vi "Parse Auto Data.vi"(10 "Is Blue Alliance?":bool=TRUE, 11 "path":path) -> (1 "Zero Velocity?":bool[](array[boolean]), 2 "Velocities":T3[](array[typedef]), 3 "Positions":cluster{"x":dbl, "y":dbl, "th":dbl}[](array[cluster]), 5 "Commands out":cluster{"Time (s)":dbl, T1, bool}[](array[cluster]), 7 "Overall":cluster{"Time (s)":dbl, "Distance (ft)":dbl})   [LabVIEW 2023]
uses:
  swerve/Type Definitions/Data/Robot Velocities.ctl
  bordeaux-pathinator/Bordeaux/Types/Single Cmd Info.ctl
  <vilib>/picture/picture.llb/imagedata.ctl
  <vilib>/Analysis/coordinate.llb/2D Cartesian Coordinate Rotation (Scalar).vi
  <vilib>/Rock Robotics/Network Tables/NT Read Boolean.vi
  <vilib>/Analysis/NI_AALPro.lvlib
panel:
  out "XY Graph":cluster{dbl[], dbl[]}[](graph)
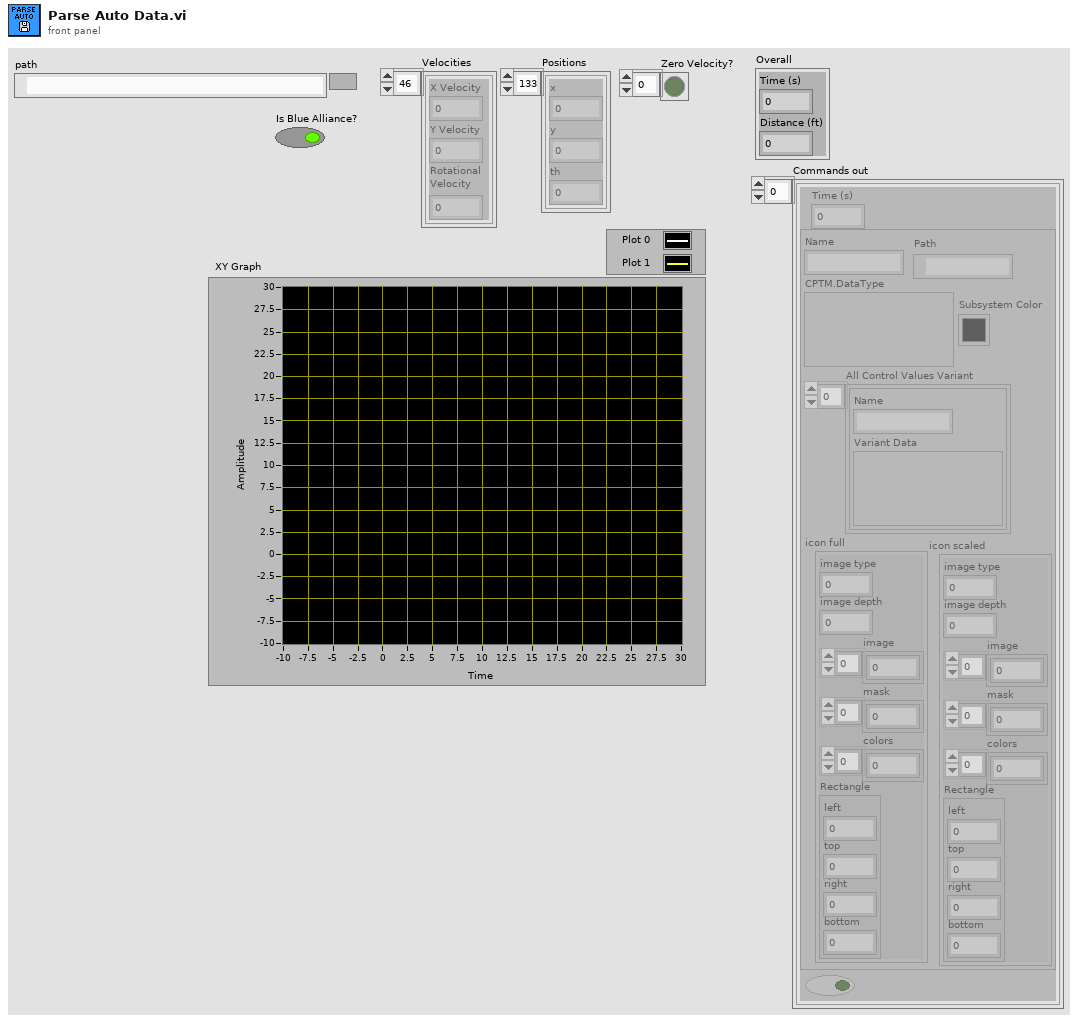
[diagram p1: front panel]
types:
  T1 = typedef "Single Cmd Info.ctl" = cluster{"Name":string, "CPTM.DataType":variant, "All Control Values Variant":cluster{"Name":string, "Variant Data":variant}[], "icon full":T2, "icon scaled":T2, "Path":path, "Subsystem Color":u32}
  T2 = typedef "imagedata.ctl" = cluster{"image type":i32, "image depth":i32, "image":u8[], "mask":u8[], "colors":u32[], "Rectangle":cluster{"left":i16, "top":i16, "right":i16, "bottom":i16}}
  T3 = typedef "Robot Velocities.ctl" = cluster{"X Velocity":dbl, "Y Velocity":dbl, "Rotational \nVelocity":dbl}
  T4 = typedef "Trajectory Data.ctl" = cluster{"Segment Name":string, "Type":T5, "Traj Pos Points":cluster{"x":dbl, "y":dbl, "th":dbl}[], "Traj Vel Points":cluster{"V":dbl, "Omega":dbl, "V vector":cluster{"y":dbl, "x":dbl}}[], "Accel Index":i32, "Decel Index":i32}[]
  T5 = typedef "Segment Type.ctl" = enum16{"Accel Straight", "Const Straight", "Blend", "Circle", "Bezier"}
  T6 = cluster{"V":dbl, "Omega":dbl, "V vector":cluster{"y":dbl, "x":dbl}}[]
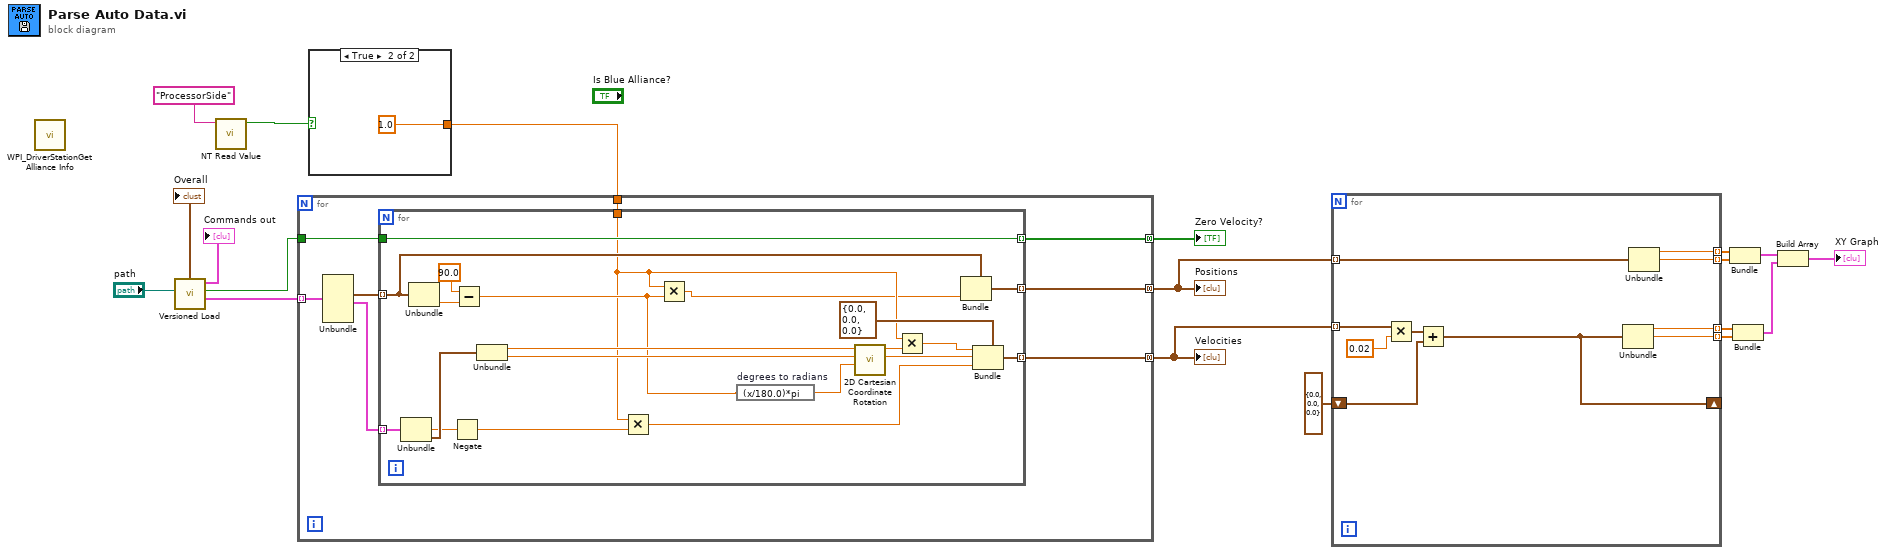
[diagram p0: block diagram]
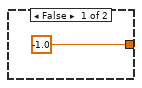
[diagram p2: hidden frame]
diagram:
  n1 = call <vilib>:"WPI_DriverStationGet Alliance Info.vi"() -> ()  [unwired: 6 in, 6 out]
  n2 = call "Versioned Load.vi"("path"="path") -> ("Trajectory Data"=w19:T4, "Zero V"=w17:bool, "Commands out"=→"Commands out":cluster{"Time (s)":dbl, T1, bool}[], "Overall"=→"Overall":cluster{"Time (s)":dbl, "Distance (ft)":dbl})  [unwired: 3 in, 4 out]
  n3 = call-poly <vilib>:"NT Read Value.vi"("name"="ProcessorSide") -> ("value"=w2:bool)  [unwired: 8 in, 2 out]
  n4 = case shown="True" w2 {
    tunnel: [-1.0 1.0] -> w18
    frame False {
    }
    frame True {
    }
  }
  n5 = for {
    tunnel: w19 -> [w29] mode=indexing
    tunnel: [w26] -> w14 mode=concatenating
    tunnel: w18 -> [w25]
    tunnel: [w22] -> w13 mode=concatenating
    tunnel: w17 -> [w24]
    tunnel: [w23] -> w16 mode=concatenating
    n6 = Unbundle(w29) -> ("Traj Pos Points"=w28:cluster{"x":dbl, "y":dbl, "th":dbl}[], "Traj Vel Points"=w27:T6)  [unwired: 4 out]
    n7 = for {
      tunnel: w28 -> [w48] mode=indexing
      tunnel: w27 -> [w46] mode=indexing
      tunnel: [w47] -> w26 mode=indexing
      tunnel: w25 -> [w31]
      tunnel: [w38] -> w22 mode=indexing
      tunnel: w24 -> [w35]
      tunnel: [w35] -> w23 mode=indexing
      n8 = Unbundle(w46) -> ("Omega"=w34:dbl, "V vector"=w45:cluster{"y":dbl, "x":dbl})  [unwired: 1 out]
      n9 = Unbundle(w48) -> ("th"=w50:dbl)  [unwired: 2 out]
      n10 = Negate(x=w34) -> (-x=w33:dbl)
      n11 = Subtract(x=90.0, y=w50) -> (x-y=w32:dbl)
      n12 = Unbundle(w45) -> ("y"=w43:dbl, "x"=w42:dbl)
      n13 = Multiply(x=w31, y=w33) -> (x*y=w40:dbl)
      n14 = Multiply(x=w31, y=w32) -> (x*y=w30:dbl)
      n15 = expression code="(x/180.0)*pi" "degrees to radians"(w32) -> (w44:dbl)
      n16 = call-poly <vilib>:"2D Cartesian Coordinate Rotation.vi"("theta"=w44, "y"=w42, "x"=w43) -> ("y out"=w41:dbl, "x out"=w37:dbl)  [unwired: 6 in, 1 out]
      n17 = Multiply(x=w31, y=w37) -> (x*y=w36:dbl)
      n18 = Bundle(cluster=w48, "th"=w30) -> (w47:cluster{"x":dbl, "y":dbl, "th":dbl})  [unwired: 2 in]
      n19 = Bundle(cluster=T3 {"X Velocity"=0.0, "Y Velocity"=0.0, "Rotational \nVelocity"=0.0} ("Robot Velocities"), "X Velocity"=w36, "Y Velocity"=w41, "Rotational \nVelocity"=w40) -> (w38:T3)
    }
  }
  "Positions" <- w14
  "Velocities" <- w13
  "Zero Velocity?" <- w16
  n20 = for {
    tunnel: w14 -> [w60] mode=indexing
    tunnel: w13 -> [w57] mode=indexing
    tunnel: [w59] -> w12 mode=indexing
    tunnel: [w58] -> w11 mode=indexing
    shift-right: [w53] -> _
    shift-left: T3 {"X Velocity"=0.0, "Y Velocity"=0.0, "Rotational \nVelocity"=0.0} ("Robot Velocities") -> [w54]
    tunnel: [w52] -> w9 mode=indexing
    tunnel: [w51] -> w8 mode=indexing
    n21 = Multiply(x=w57, y=0.02) -> (x*y=w55:T3)
    n22 = Add(x=w55, y=w54) -> (x+y=w53:T3)
    n23 = Unbundle(w53) -> ("X Velocity"=w52:dbl, "Y Velocity"=w51:dbl)  [unwired: 1 out]
    n24 = Unbundle(w60) -> ("x"=w59:dbl, "y"=w58:dbl)  [unwired: 1 out]
  }
  n25 = Bundle(w12, w11) -> (w7:cluster{dbl[], dbl[]})  [unwired: 1 in]
  n26 = Bundle(w9, w8) -> (w6:cluster{dbl[], dbl[]})  [unwired: 1 in]
  n27 = Build Array(w7, w6) -> (→"XY Graph":cluster{dbl[], dbl[]}[])
